vi "Blue Indicator.vi"() -> (1 "Color":T1=20)   [LabVIEW 2019]
uses:
  Indicator LED - Blue.ctl
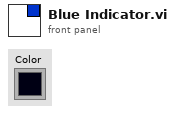
[diagram p1: front panel]
types:
  T1 = typedef "Indicator LED - Blue.ctl" = u32
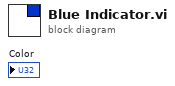
[diagram p0: block diagram]
diagram:
